vi "CR-导丝上料一致性处理函数.vi"(8 "error in (no error)":errorcluster caption="错误输入（无错误）", 9 "导丝上料一致性参数":T6={"Rectangle"={"Left"=0, "Top"=0, "Right"=0, "Bottom"=0, "Rotation"=0.0}, "Find Straight Edge 1"={"Number of Lines"=1, "Type"=enum."First Edge Rake", "Min. Score"=10.0, "Max. Score"=1000.0, "Orientation"=0.0, "Angle Range"=45.0, "Angle Tolerance"=1.0, "Step Size"=11, "Min. SNR (db)"=0.0, "Min. Points (%)"=25.0, "Hough Iterations"=5}, "Process (Edge Detector 1)"=enum."Get All Edges", "Edge Options (Edge Detector 1)"={"Edge Polarity"=0, "Kernel Size"=9, "Width"=1, "Minimum Edge Strength"=8.0, "Interpolation Type"=enum."Bilinear Fixed", "Data Processing Method"=enum."Average"}, "Options (Find Straight Edge 1)"={"Search Direction"=0, "Edge Options"={"Edge Polarity"=0, "Kernel Size"=3, "Width"=1, "Minimum Edge Strength"=32.0, "Interpolation Type"=enum."Bilinear Fixed", "Data Processing Method"=enum."Average"}, "Show Search Area"=TRUE, "Show Search Lines"=TRUE, "Show Edges Found"=TRUE, "Show Result"=TRUE, "Search Area Color"=65280, "Search Lines Color"=255, "Edge Locations Color"=16776960, "Result Color"=16711680, "Overlay Group Name"=""}, "Parameters (Pattern Matching 1)"={"Number of Matches Requested"=1, "Minimum Match Score"=799.0, "Angle Ranges"=[{"Start Angle"=-180.0, "End Angle"=180.0}, {"Start Angle"=0.0, "End Angle"=360.0}]}, "Template File Path (Pattern Matching 1)"=path "D:/Inspect System/Source Code/Template Program/一致性模板.png"} {"Options (Find Straight Edge 1)"."Search Direction" items=["Left to Right", "Right to Left", "Top to Bottom", "Bottom to Top"]; "Options (Find Straight Edge 1)"."Edge Options"."Edge Polarity" items=["All Edges", "Rising Edges", "Falling Edges"]; "Options (Find Straight Edge 1)"."Edge Options"."Minimum Edge Strength" format="%.2f"; "Options (Find Straight Edge 1)"."Edge Options"."Width" step=2; "Options (Find Straight Edge 1)"."Edge Options"."Kernel Size" step=2; "Edge Options (Edge Detector 1)"."Edge Polarity" items=["All Edges", "Rising Edges", "Falling Edges"]; "Find Straight Edge 1"."Min. Points (%)" min=0.0 max=100.0; "Find Straight Edge 1"."Min. SNR (db)" min=0.0; "Find Straight Edge 1"."Max. Score" min=0.0 max=1024.0; "Find Straight Edge 1"."Min. Score" min=0.0 max=1024.0 step=1.0; "Rectangle"."Rotation" format="%.2f"; "Rectangle"."Left" scale=0.0..1024.0; "Rectangle"."Right" scale=0.0..1024.0}, 10 "位置范围设定":T7={"位置1"={"上限"=726.0, "下限"=686.0}, "位置2"={"上限"=874.0, "下限"=834.0}, "位置3"={"上限"=997.0, "下限"=957.0}, "位置4"={"上限"=1139.0, "下限"=1099.0}, "位置5"={"上限"=1283.0, "下限"=1243.0}, "位置6"={"上限"=1429.0, "下限"=1389.0}, "位置7"={"上限"=1576.0, "下限"=1536.0}, "位置8"={"上限"=1728.0, "下限"=1688.0}, "位置9"={"上限"=1879.0, "下限"=1839.0}, "位置10"={"上限"=2036.0, "下限"=1996.0}}, 11 "Image in":T8(plugin-control)) -> (0 "error out":errorcluster caption="错误输出", 1 "动态范围":sgl[](array[numeric]), 2 "一致性结果字符串":string, 3 "Image out":T8(plugin-control))   [LabVIEW 2017]
uses:
  <vilib>/vision/Measure.llb/Straight Edge Options.ctl
  <vilib>/vision/Measure.llb/Straight Edge Process.ctl
  <vilib>/vision/Measure.llb/Edge Options.ctl
  <vilib>/vision/Measure.llb/Edge Polarity.ctl
panel:
  out "字符串":string
  out "反转 2":string
  out "反转":string
  out "子字符串 2":string
  out "子字符串":string
  # "0000101000"
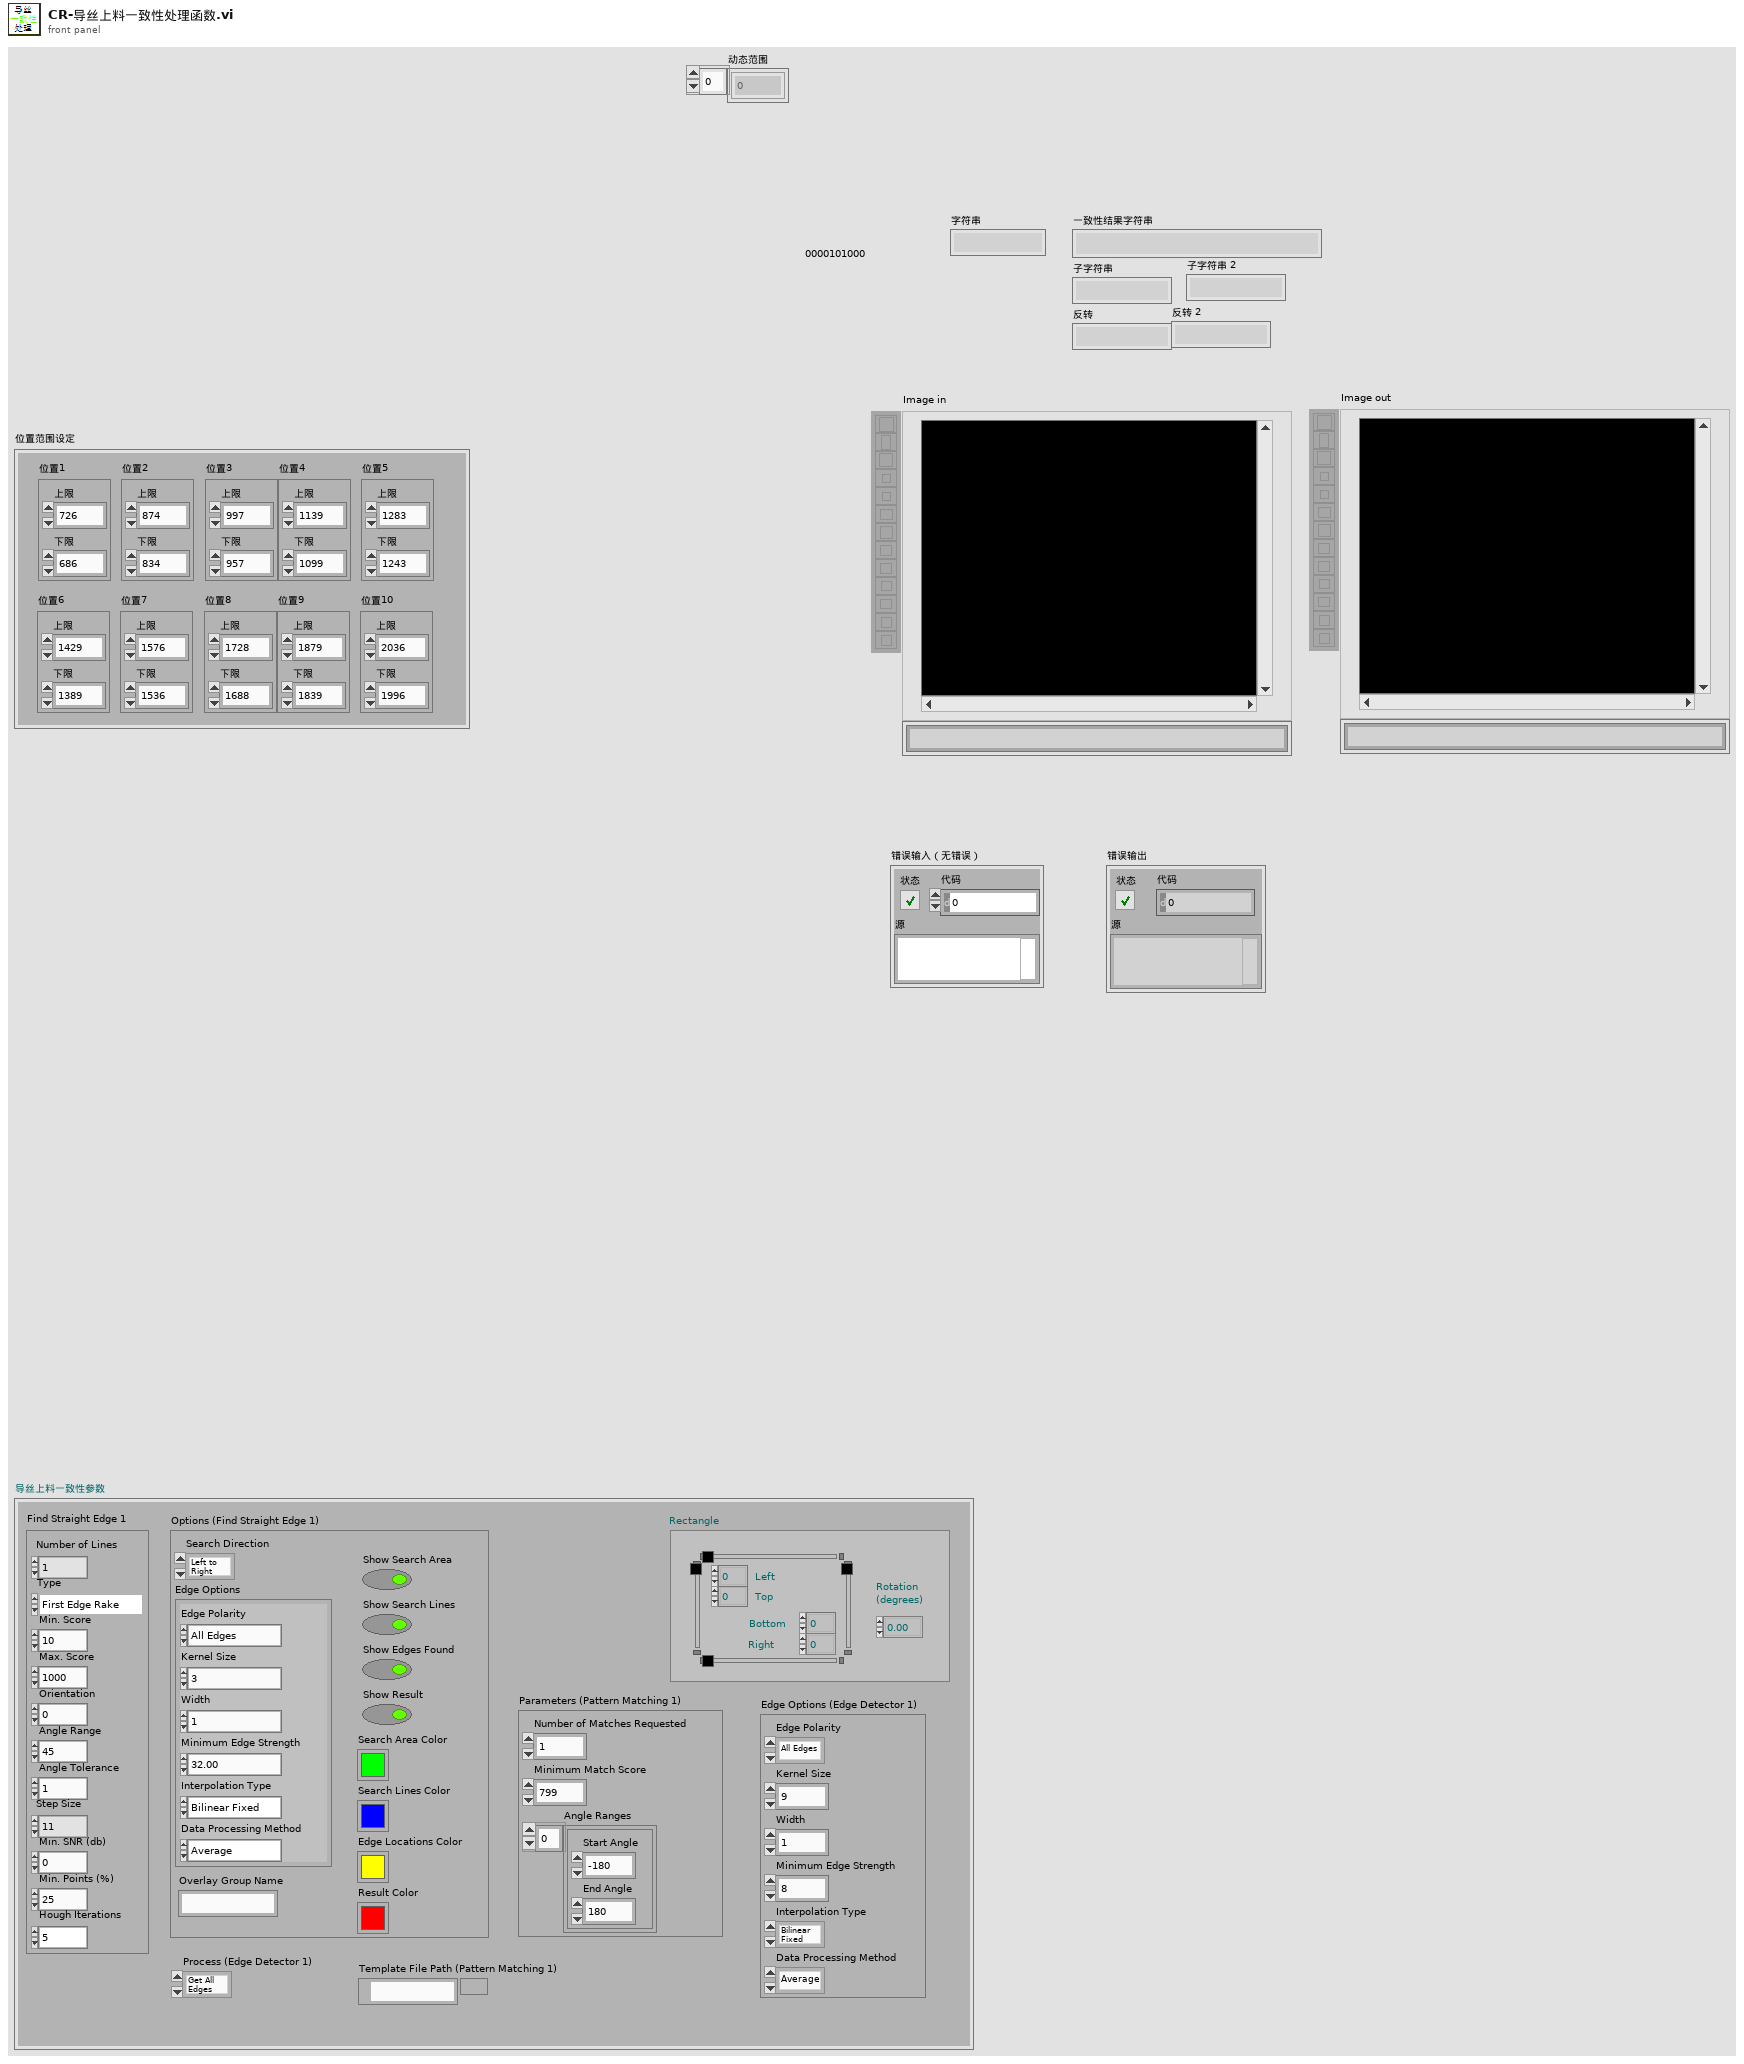
[diagram p1: front panel]
types:
  T1 = typedef "IMAQ Rectangle" = cluster{"Left":i32, "Top":i32, "Right":i32, "Bottom":i32, "Rotation":dbl}
  T2 = typedef "Straight Edge Options.ctl" = cluster{"Number of Lines":i32, "Type":T3, "Min. Score":dbl, "Max. Score":dbl, "Orientation":dbl, "Angle Range":dbl, "Angle Tolerance":dbl, "Step Size":u32, "Min. SNR (db)":dbl, "Min. Points (%)":dbl, "Hough Iterations":i32}
  T3 = typedef "Straight Edge Process.ctl" = enum32{"First Edge Rake", "Best Edge Rake", "Hough Edge Rake", "First Edge Projection", "Best Edge Projection"}
  T4 = typedef "Edge Options.ctl" = cluster{"Edge Polarity":T5, "Kernel Size":u32, "Width":u32, "Minimum Edge Strength":sgl, "Interpolation Type":enum32{"Zero Order", "Bilinear", "Quadratic", "Cubic", "Bilinear Fixed"}, "Data Processing Method":enum32{"Average", "Median"}}
  T5 = typedef "Edge Polarity.ctl" = u32
  T6 = cluster{"Rectangle":T1, "Find Straight Edge 1":T2, "Process (Edge Detector 1)":enum16{"Get First Edge", "Get First + Last Edge", "Get All Edges", "Get Best Edge"}, "Edge Options (Edge Detector 1)":cluster{"Edge Polarity":u32, "Kernel Size":u32, "Width":u32, "Minimum Edge Strength":sgl, "Interpolation Type":enum32{"Zero Order", "Bilinear", "Quadratic", "Cubic", "Bilinear Fixed"}, "Data Processing Method":enum32{"Average", "Median"}}, "Options (Find Straight Edge 1)":cluster{"Search Direction":u32, "Edge Options":T4, "Show Search Area":bool, "Show Search Lines":bool, "Show Edges Found":bool, "Show Result":bool, "Search Area Color":u32, "Search Lines Color":u32, "Edge Locations Color":u32, "Result Color":u32, "Overlay Group Name":string}, "Parameters (Pattern Matching 1)":cluster{"Number of Matches Requested":i32, "Minimum Match Score":sgl, "Angle Ranges":cluster{"Start Angle":sgl, "End Angle":sgl}[]}, "Template File Path (Pattern Matching 1)":path}
  T7 = cluster{"位置1":cluster{"上限":dbl, "下限":dbl}, "位置2":cluster{"上限":dbl, "下限":dbl}, "位置3":cluster{"上限":dbl, "下限":dbl}, "位置4":cluster{"上限":dbl, "下限":dbl}, "位置5":cluster{"上限":dbl, "下限":dbl}, "位置6":cluster{"上限":dbl, "下限":dbl}, "位置7":cluster{"上限":dbl, "下限":dbl}, "位置8":cluster{"上限":dbl, "下限":dbl}, "位置9":cluster{"上限":dbl, "下限":dbl}, "位置10":cluster{"上限":dbl, "下限":dbl}}
  T8 = typedef "IMAQ Image.ctl" = refnum<image>
  T9 = cluster{"Desired Font (Application)":enum16{"User-specified Font", "Application Font", "System Font", "Dialog Font"}, "[User-specified Font]":cluster{"Font Name":string, "Size":i16, "Strikeout?":bool, "Italic?":bool, "Underline?":bool, "Outline?":bool, "Shadow?":bool, "Bold?":bool, "Rotation Angle":dbl}, "Horizontal Alignment":i16, "Vertical Alignment":i16}
  T10 = typedef "Image Type" = u32
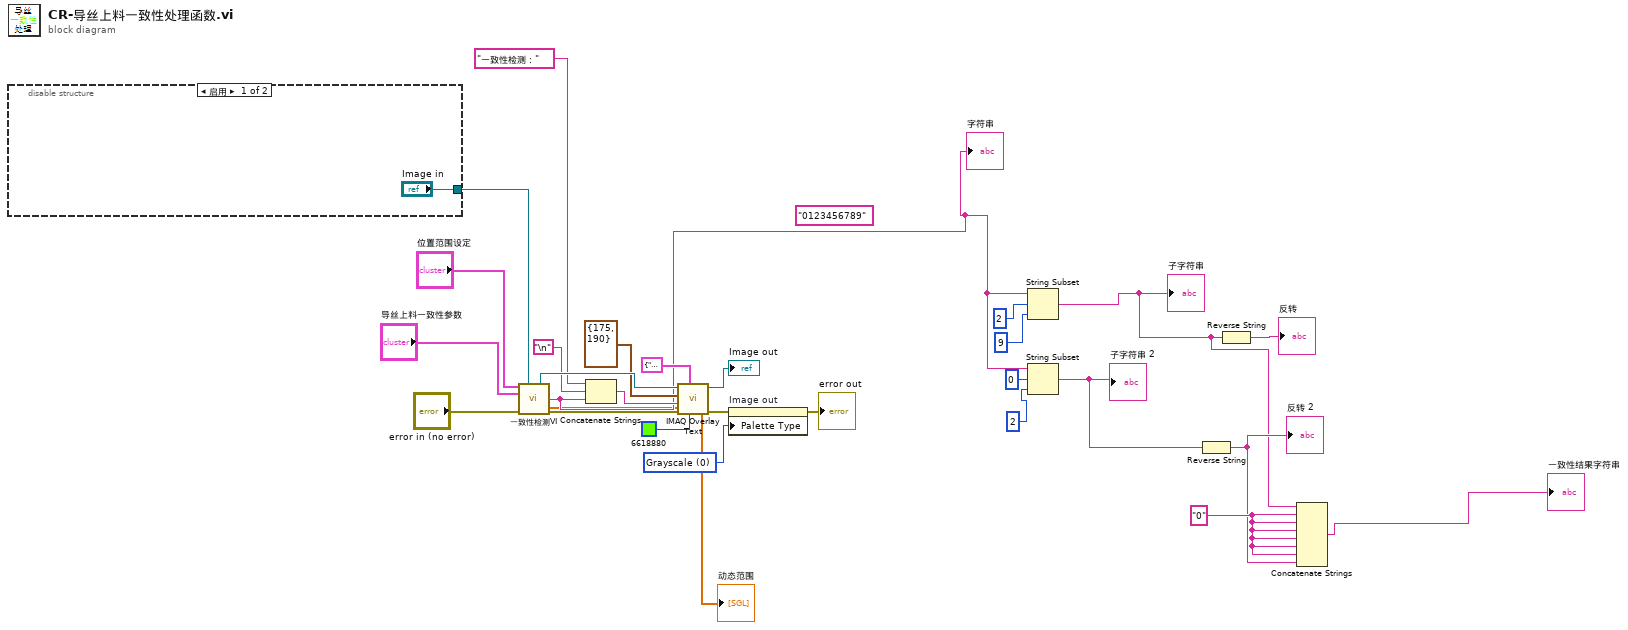
[diagram p0: block diagram]
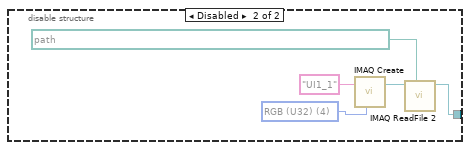
[diagram p2: hidden frame]
diagram:
  w8 = "0" ("字符串")
  (unwired) "0123456789" ("一致性结果字符串")
  w28 = u32 0 items=["Grayscale", "Binary", "Gradient", "Rainbow", "Temperature", "User Defined", "Binary 16 Bit", "Gradient 16 Bit", "Rainbow 16 Bit", "Temperature 16 Bit", "User Defined 16 Bit"] ("Palette:Palette Type")
  n1 = disable-structure shown="启用" {
    disable-tunnel: ["Image in" w30] -> w27
    frame Enabled {
    }
    frame Disabled {
      w33 = T10 4 items=["Grayscale (U8)", "Grayscale (I16)", "Grayscale (SGL)", "Complex (CSG)", "RGB (U32)", "HSL (U32)", "RGB (U64)", "Grayscale (U16)"] ("Image Type")
      n2 = call "IMAQ Create"("Image Name"="UI1_1", "Image Type"=w33) -> ("New Image"=w32:T8)  [unwired: 3 in, 1 out]
      n3 = call "IMAQ ReadFile 2"("File Path"=path "D:/Inspect System/Source Code/SubVIs/衬丝检测/衬丝3.png", "Image"=w32) -> ("Image Out"=w30:T8)  [unwired: 5 in, 4 out]
    }
  }
  n4 = call "一致性检测VI.vi"("位置范围设定"="位置范围设定", "Image in"=w27, "导丝上料一致性参数"="导丝上料一致性参数", "error in (no error)"="error in (no error)") -> ("Image out"=w22:T8, "字符串"=w3:string, "动态范围"=→"动态范围":sgl[], "error out"=w19:errorcluster)  [unwired: 5 in, 3 out]
  "字符串" <- w3
  n5 = Concatenate Strings("一致性检测：" ("字符串"), "\n", w3) -> (w13:string)
  n6 = call "IMAQ Overlay Text"("Text Color (black)"=u32 6618880, "Font, Size & Style"=T9 {"Desired Font (Application)"=enum."User-specified Font", "[User-specified Font]"={"Font Name"="", "Size"=200, "Strikeout?"=FALSE, "Italic?"=FALSE, "Underline?"=FALSE, "Outline?"=FALSE, "Shadow?"=TRUE, "Bold?"=TRUE, "Rotation Angle"=0.0}, "Horizontal Alignment"=0, "Vertical Alignment"=0}, "error in (no error)"=w19, "String"=w13, "Origin"=cluster{"X":i32, "Y":i32} {"X"=175, "Y"=190}, "Image"=w22) -> ("error out"=w18:errorcluster, "Image Out"=→"Image out":T8)  [unwired: 4 in]
  n7 = property on="Image out" class="ImageControl"(error in=w18, "Palette Type"=w28) -> (error out=→"error out":errorcluster)  [unwired: 1 in, 1 out]
  n8 = String Subset(string=w3, offset (0)=2 ("偏移量(0)"), length (rest)=9 ("长度（剩余）")) -> (substring=w2:string)
  "子字符串" <- w2
  n9 = String Subset(string=w3, offset (0)=0 ("偏移量(0)"), length (rest)=2 ("长度（剩余）")) -> (substring=w9:string)
  "子字符串 2" <- w9
  n10 = Reverse String(1:w9) -> (0:w7:string)
  "反转 2" <- w7
  n11 = Reverse String(1:w2) -> (0:→"反转":string)
  n12 = Concatenate Strings(w2, w8, w8, w8, w8, w8, w8, w7) -> (→"一致性结果字符串":string)
